vi "Rozbicie tekstu na współrzędną w formacie DM.vi"(7 "Współrzędna tekstowa":string) -> (0 "Kierunek":string, 1 "Druga współrzędna":string, 3 "M":dbl, 5 "D":dbl)   [LabVIEW 2015, in "Biblioteka moduł map v3.lvlib" / "Konwersja wsp.lvlib" / "Wyciągnięcie z tekstu współrzędnej.lvlib"]
doc: "SubVI ma za zadanie odfiltrować pierwszą współrzędną. Podaje jej stopnie i minuty jako liczbę double oraz kierunek geograficzny. Dodatkowo jest możliwość dalszego odfiltrowania tekstu i odfiltrowanie kolejnej współrzędnej."
uses:
  <vilib>/regexp/Match Regular Expression.xnode
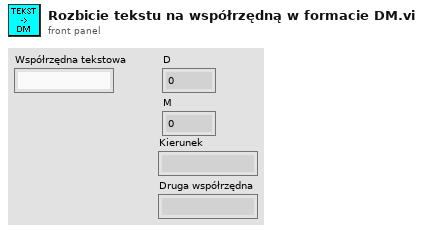
[diagram p1: front panel]
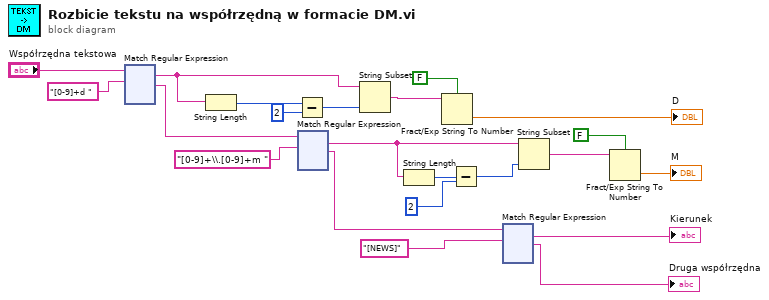
[diagram p0: block diagram]
diagram:
  n1 = xnode "Match Regular Expression"("input string"="Współrzędna tekstowa", "regular expression"="[0-9]+d ") -> ("whole match"=w3:string, "after match"=w4:string)  [unwired: 4 in, 3 out]
  n2 = String Length(string=w3) -> (length=w10:i32)
  n3 = Subtract(x=w10, y=2) -> (x-y=w8:i32)
  n4 = xnode "Match Regular Expression"("input string"=w4, "regular expression"="[0-9]+\\.[0-9]+m ") -> ("whole match"=w12:string, "after match"=w16:string)  [unwired: 4 in, 3 out]
  n5 = String Subset(string=w3, length (rest)=w8) -> (substring=w17:string)  [unwired: 1 in]
  n6 = String Length(string=w12) -> (length=w5:i32)
  n7 = Fract/Exp String To Number(use system decimal point (T)=FALSE, string=w17) -> (number=→"D":dbl)  [unwired: 2 in, 1 out]
  n8 = Subtract(x=w5, y=2) -> (x-y=w7:i32)
  n9 = xnode "Match Regular Expression"("input string"=w16, "regular expression"="[NEWS]") -> ("whole match"=→"Kierunek":string, "after match"=→"Druga współrzędna":string)  [unwired: 4 in, 3 out]
  n10 = String Subset(string=w12, length (rest)=w7) -> (substring=w14:string)  [unwired: 1 in]
  n11 = Fract/Exp String To Number(use system decimal point (T)=FALSE, string=w14) -> (number=→"M":dbl)  [unwired: 2 in, 1 out]
